vi "Comm GV.vi"() -> ()   [LabVIEW 2019, in "Shared.lvlib"]
uses:
  Shared.lvlib
  Intertarget communication/Command + data + response cluster.ctl
  Intertarget communication/Status + response + data cluster.ctl
  Data message cluster.ctl
  mmWave data_class/mmWave data.lvclass
  Error event data.ctl
  Intertarget communication/CommandResponse communication.lvlib
panel:
  in  "Error":refnum<user-event>
  in  "NewData":refnum<user-event>
  in  "CloseApp":refnum<user-event>
  in  "Command":refnum<user-event>
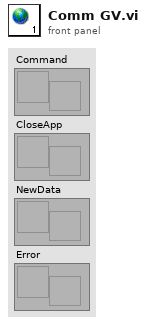
[diagram p1: front panel]
diagram:
